vi "ConverteixAD.vi"(1 "ValorSenseTara":refnum<vi>, 7 "ValorAdquirid":dbl, 9 "Unitats":refnum<vi>, 10 "Tara":refnum<vi>, 11 "FactorsUnitatsPendents":refnum<vi>) -> (0 "Escala":u8, 2 "ValorActualAbs":dbl, 3 "ValorSenseTara":dbl)   [LabVIEW 2017]
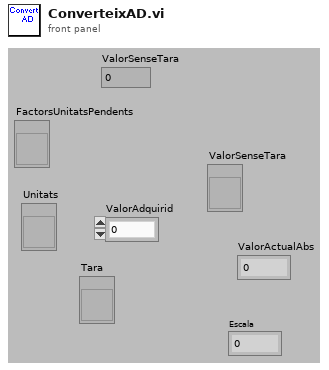
[diagram p1: front panel]
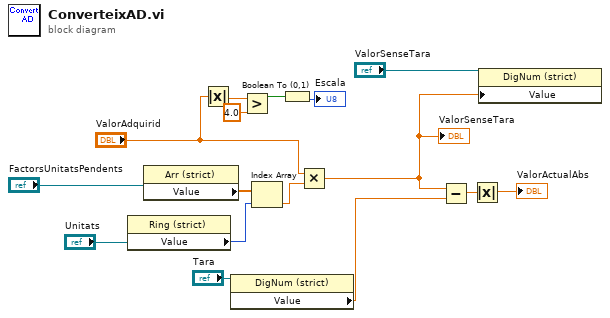
[diagram p0: block diagram]
diagram:
  n1 = property class="Ring (strict)"(reference="Unitats") -> ("Value"=w13:u16)  [unwired: 1 in, 2 out]
  n2 = property class="Arr (strict)"(reference="FactorsUnitatsPendents") -> ("Value"=w14:dbl[])  [unwired: 1 in, 2 out]
  n3 = Absolute Value(x="ValorAdquirid") -> (abs(x)=w2:dbl)
  n4 = property class="DigNum (strict)"(reference="Tara") -> ("Value"=w10:sgl)  [unwired: 1 in, 2 out]
  n5 = Greater?(x=w2, y=4.0) -> (0:w4:bool)
  n6 = Index Array(array=w14, index=w13) -> (element=w12:dbl)
  n7 = Boolean To (0,1)(Boolean=w4) -> (0, 1=→"Escala":i16)
  n8 = Multiply(x="ValorAdquirid", y=w12) -> (x*y=w8:dbl)
  "ValorSenseTara" <- w8
  n9 = Subtract(x=w8, y=w10) -> (x-y=w7:dbl)
  n10 = Absolute Value(x=w7) -> (abs(x)=→"ValorActualAbs":dbl)
  n11 = property class="DigNum (strict)"(reference="ValorSenseTara", "Value"=w8) -> ()  [unwired: 1 in, 2 out]
